vi "ziGetValueDIO.vi"(3 "error in":errorcluster, 4 "Path":string, 5 "Handle In":T1 {"Handle" format="0x%08x"; "Conn" format="0x%08x"}) -> (0 "error out":errorcluster, 1 "DIO Value":cluster{"dt (ticks)":u64, "value":u32}, 2 "Handle Out":T1 {"Handle" format="0x%08x"; "Conn" format="0x%08x"})   [LabVIEW 2018, in "Zurich Instruments LabOne.lvlib"]
doc: "This vi retrieves the newest available DIO sample from the specified node. The vi returns the value first found if more than one value is available (a wildcard is used in the Path). This function is only applicable to nodes ending in \"DIOS/[0-9]+/input\"."
uses:
  Zurich Instruments LabOne.lvlib
  <instrlib>/Zurich Instruments LabOne/Private/ziLV64.framework
  ziTypeHandle.ctl
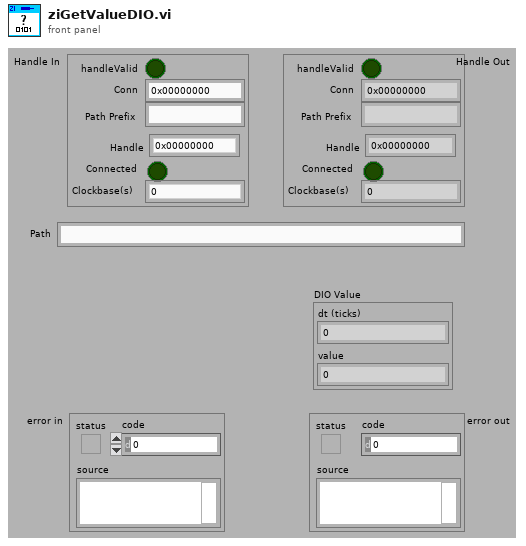
[diagram p1: front panel]
types:
  T1 = typedef "Zurich Instruments LabOne.lvlib/ziTypeHandle.ctl" = cluster{"handleValid":bool, "Conn":u64, "Path Prefix":string, "Handle":u64, "Connected":bool, "Clockbase(s)":dbl}
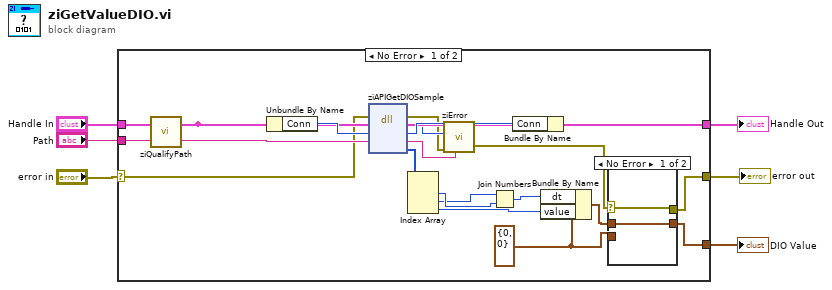
[diagram p0: block diagram]
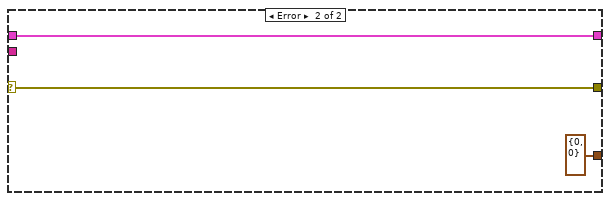
[diagram p3: hidden frame]
diagram:
  n1 = case shown="No Error" "error in" {
    selector: "error in" -> [w15 w34]
    tunnel: [w27 w33] -> w6
    tunnel: [w12 cluster{"dt":u64, "value":u32} {"dt"=0, "value"=0} ("DioVal")] -> w5
    tunnel: "Path" -> [w20 _]
    tunnel: "Handle In" -> [w19 w33]
    tunnel: [w9 w34] -> w2
    frame No Error {
      w11 = cluster{"dt":u64, "value":u32} {"dt"=0, "value"=0} ("DioVal")
      n2 = call "ziQualifyPath.vi"("Path In"=w20, "Handle In"=w19) -> ("Path Out"=w21:string, "Handle Out"=w22:T1)
      n3 = Unbundle By Name(w22) -> ("Conn"=w26:u64)
      n4 = dll-call lib="Applications/National Instruments/LabVIEW 2019 64-bit/instr.lib/Zurich Instruments LabOne/Private/ziLV*.*" fn="ziAPIGetDIOSample" label="ziAPIGetValueDIO"(error in=w15, "Conn"=w26, "Path"=w21) -> (error out=w16:errorcluster, "return type"=w18:u32, "Conn"=w25:u64, "Path"=w14:string, "DIOSample"=w24:u32[])  [unwired: 2 in, 2 out]
      n5 = Index Array(array=w24) -> (element #1=w8:u32, element #2=w7:u32, element #3=w23:u32)  [unwired: 3 in]
      n6 = call "ziError.vi"("ziErrorCode"=w18, "Error In"=w16, "Annotation"=w14) -> ("Error Out"=w10:errorcluster)  [unwired: 3 in]
      n7 = Join Numbers(hi=w7, lo=w8) -> ((hi.lo)=w17:u64)
      n8 = Bundle By Name(cluster=w22, "Conn"=w25) -> (w27:T1)
      n9 = Bundle By Name(cluster=w11, "dt"=w17, "value"=w23) -> (w13:cluster{"dt":u64, "value":u32})
      n10 = case shown="No Error" w10 {
        selector: w10 -> [w28 w30]
        tunnel: w13 -> [w29 _]
        tunnel: [w29 w31] -> w12
        tunnel: w11 -> [_ w31]
        tunnel: [w28 w30] -> w9
        frame No Error {
        }
        frame Error {
        }
      }
    }
    frame Error {
    }
  }
  "Handle Out" <- w6
  "error out" <- w2
  "DIO Value" <- w5
